vi "I16ToU8.vi"(5 "Number":i16) -> (1 "Unsigned 8-bit integer":u8, 2 "Overflow?":bool, 3 "Exact conversion?":bool)   [LabVIEW 2017, in "GPOverflow.lvlib"]
doc: "Converts <B>Number</B> to U8 keeping track of numeric overflow and exactness of conversion.\n\n<B>Exact conversion?</B> will be True only if a conversion back into the original data type of <B>Number</B> will yield the exact same number, i.e. no precision was lost during the conversion.\n\n<B>Overflow?</B> will be True if positive or negative overflow occurred. The numeric output will saturate in case of overflow.\n\nThis VI is inlined.\n\nSteen Schmidt\nGPower\n6/3 2013"
uses:
  GPOverflow.lvlib
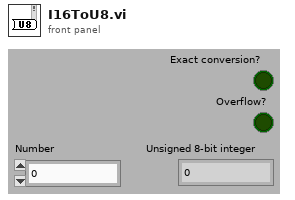
[diagram p1: front panel]
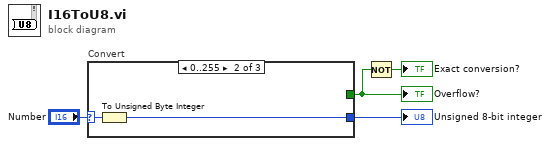
[diagram p0: block diagram]
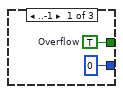
[diagram p2: hidden frame]
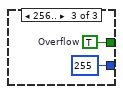
[diagram p3: hidden frame]
diagram:
  n1 = case "Convert" shown="0..255" "Number" {
    selector: "Number" -> [_ w8 _]
    tunnel: [u8 0 w7 u8 255] -> w3
    tunnel: [w5 _ w9] -> w2
    frame ..-1 {
      w5 = TRUE  # Overflow
    }
    frame 0..255 {
      n2 = To Unsigned Byte Integer(number=w8) -> (unsigned 8bit integer=w7:u8)
    }
    frame 256.. {
      w9 = TRUE  # Overflow
    }
  }
  "Unsigned 8-bit integer" <- w3
  "Overflow?" <- w2
  n3 = Not(x=w2) -> (.not. x?=→"Exact conversion?":bool)
